vi "XVA-DSE6-dist.vi"(8 "err in":errorcluster, 10 "X-VA (e)":T2, 11 "p_LExp":T1) -> (0 "err out":errorcluster, 2 "VA (s)":T2, 3 "p_LExp (s)":T1)   [LabVIEW 2010, in "lv_04.lvlib"]
uses:
  lv_04.lvlib
  commandes/cX.ctl
  commandes/cSTA_varid.ctl
  commandes/c_TDMS_ch_variable.ctl
  commandes/c_TDMS_ch_donnees.ctl
  commandes/c0-var-n.ctl
  commandes/cSTA_num_do_cr.ctl
  commandes/c02-do-num.ctl
  commandes/c04-stat-num.ctl
  commandes/cSTA_txt_do_cr.ctl
  commandes/c02-do-txt.ctl
  commandes/c04-stat-txt.ctl
  commandes/cSTA_dist.ctl
  commandes/c03-dist-S.ctl
  commandes/c0-dist-xy.ctl
  commandes/c03-dist-T.ctl
  commandes/c03-dist-SPC.ctl
  lv_02/p_5E6_Lexp.ctl
  lv_02/p_5E7_LW.ctl
  lv_02/lv_02.lvlib
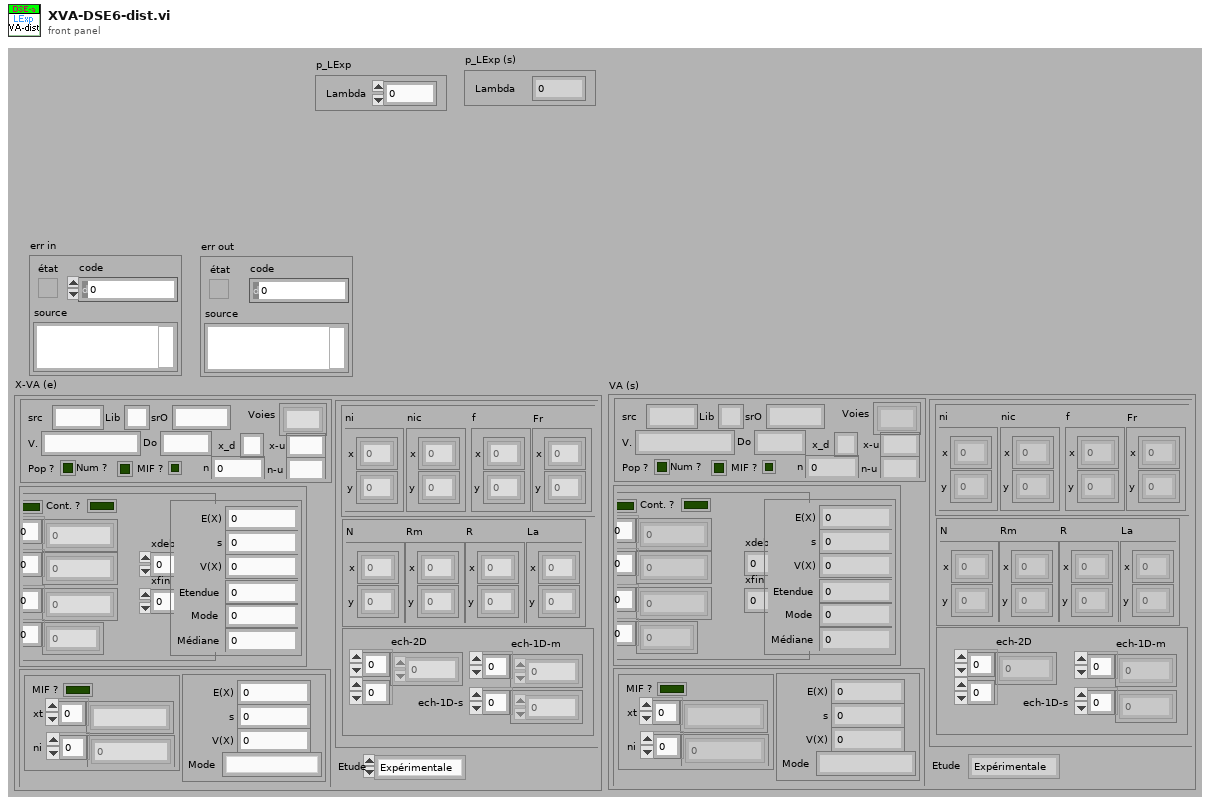
[diagram p1: front panel]
types:
  T1 = typedef "lv_02.lvlib/p_5E6_Lexp.ctl" = cluster{"Lambda":dbl}
  T2 = typedef "lv_04.lvlib/cX.ctl" = cluster{"src":T3, "num":T7, "txt":T10, "dist":T13, "Etude":enum16{"Expérimentale", "Modèle"}}
  T3 = typedef "lv_04.lvlib/cSTA_varid.ctl" = cluster{"src":string, "Lib":string, "srO":string, "V.":T4, "Voies":string[], "Do":T5, "n":T6, "Num ?":bool, "Pop ?":bool, "x_d":string, "x-u":string, "n-u":string, "MIF ?":bool}
  T4 = typedef "lv_04.lvlib/c_TDMS_ch_variable.ctl" = string
  T5 = typedef "lv_04.lvlib/c_TDMS_ch_donnees.ctl" = string
  T6 = typedef "lv_04.lvlib/c0-var-n.ctl" = i32
  T7 = typedef "lv_04.lvlib/cSTA_num_do_cr.ctl" = cluster{"do":T8, "sta":T9}
  T8 = typedef "lv_04.lvlib/c02-do-num.ctl" = cluster{"MIF ?":bool, "Cont. ?":bool, "xi":dbl[], "xic":dbl[], "ni":u32[], "dx":dbl[], "xdeb":dbl, "xfin":dbl}
  T9 = typedef "lv_04.lvlib/c04-stat-num.ctl" = cluster{"E(X)":dbl, "s":dbl, "V(X) ":dbl, "Etendue":dbl, "Mode":dbl, "Médiane":dbl}
  T10 = typedef "lv_04.lvlib/cSTA_txt_do_cr.ctl" = cluster{"do":T11, "sta":T12}
  T11 = typedef "lv_04.lvlib/c02-do-txt.ctl" = cluster{"xt":string[], "ni":dbl[], "MIF ?":bool}
  T12 = typedef "lv_04.lvlib/c04-stat-txt.ctl" = cluster{"E(X)":dbl, "s":dbl, "V(X) ":dbl, "Mode":string}
  T13 = typedef "lv_04.lvlib/cSTA_dist.ctl" = cluster{"S":T14, "T":T16, "spc":T17}
  T14 = typedef "lv_04.lvlib/c03-dist-S.ctl" = cluster{"nic":T15, "f":T15, "Fr":T15, "ni":T15}
  T15 = typedef "lv_04.lvlib/c0-dist-xy.ctl" = cluster{"x":dbl[], "y":dbl[]}
  T16 = typedef "lv_04.lvlib/c03-dist-T.ctl" = cluster{"N":T15, "Rm":T15, "R":T15, "La":T15}
  T17 = typedef "lv_04.lvlib/c03-dist-SPC.ctl" = cluster{"ech-2D":dbl[][], "ech-1D-m":dbl[], "ech-1D-s":dbl[]}
  T18 = typedef "lv_02.lvlib/p_5E7_LW.ctl" = cluster{"Beta":dbl, "Eta":dbl, "Gama":dbl}
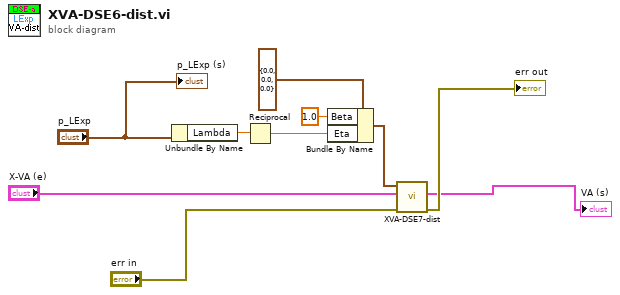
[diagram p0: block diagram]
diagram:
  n1 = Unbundle By Name("p_LExp") -> ("Lambda"=w7:dbl)
  n2 = Reciprocal(x=w7) -> (1/x=w6:dbl)
  n3 = Bundle By Name(cluster=T18 {"Beta"=0.0, "Eta"=0.0, "Gama"=0.0} ("Weibull (paramètres)"), "Beta"=1.0, "Eta"=w6) -> (w5:T18)
  n4 = call "XVA-DSE7-dist.vi"("err in"="err in", "X-VA (e)"="X-VA (e)", "p_LW"=w5) -> ("err out"=→"err out":errorcluster, "VA (s)"=→"VA (s)":T2)  [unwired: 6 in, 1 out]
  "p_LExp (s)" <- "p_LExp"
